vi "calc_drift.vi"(8 "error in (no error)":errorcluster caption="错误输入（无错误）", 11 "OneMotion 输入":refnum<class "OneMotion.lvclass">) -> (0 "error out":errorcluster caption="错误输出", 3 "OneMotion 输出":refnum<class "OneMotion.lvclass">)   [LabVIEW 2014, in "OneMotion.lvclass"]
uses:
  OneMotion.lvclass
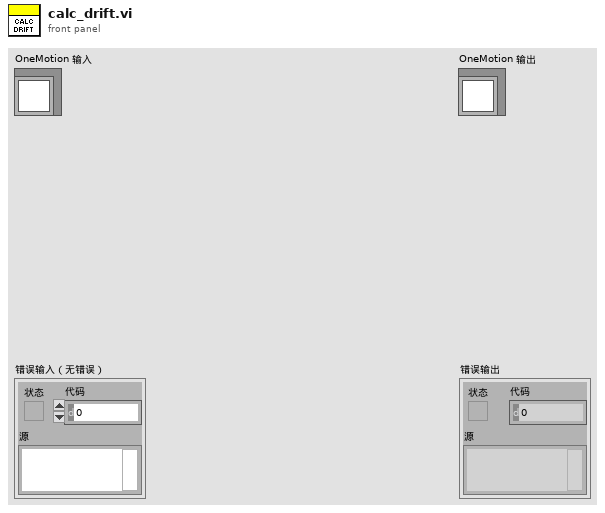
[diagram p1: front panel]
types:
  T1 = typedef "OneMotion.lvclass/backlash option.ctl" = enum16{"no backlash compensation", "compensation: from - to +", "compensation: from + to -"}
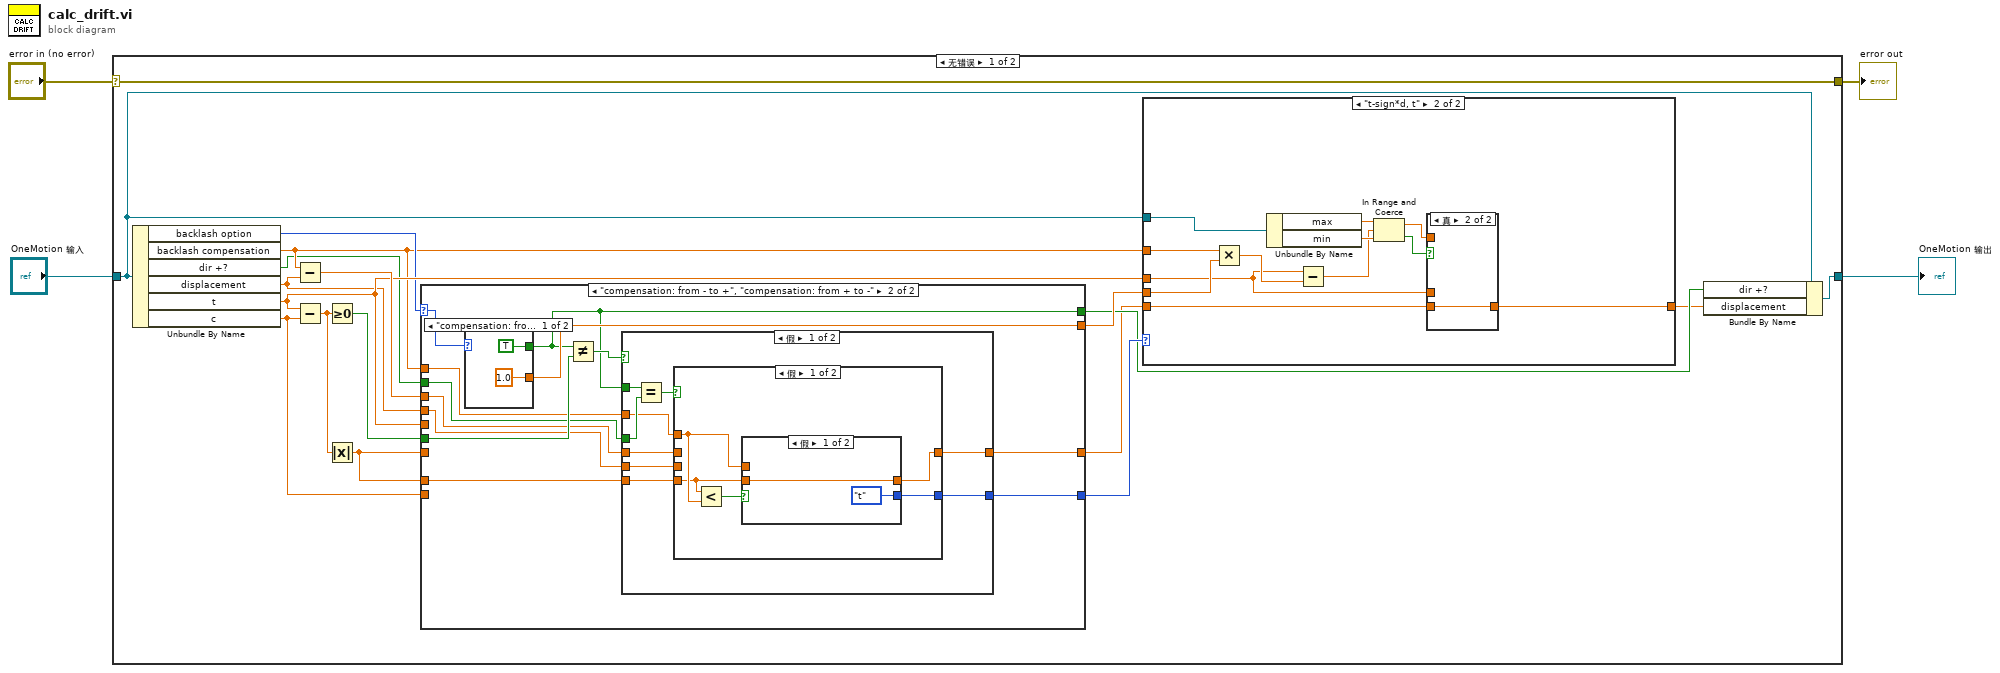
[diagram p0: block diagram]
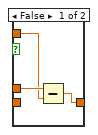
[diagram p3: hidden frame]
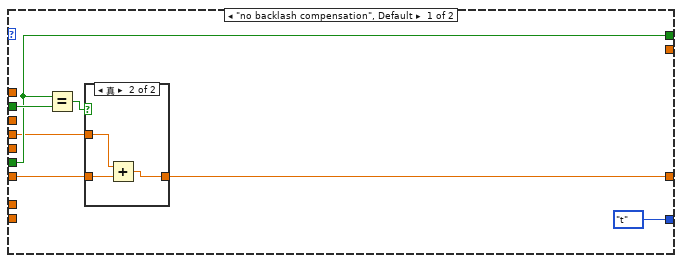
[diagram p4: hidden frame]
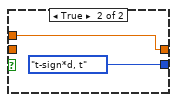
[diagram p6: hidden frame]
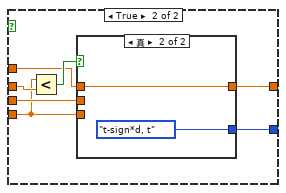
[diagram p7: hidden frame]
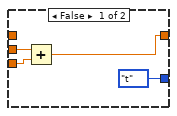
[diagram p8: hidden frame]
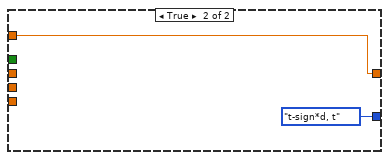
[diagram p9: hidden frame]
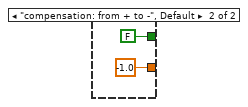
[diagram p10: hidden frame]
diagram:
  n1 = case shown="无错误" "error in (no error)" {
    selector: "error in (no error)" -> [w22 w101]
    tunnel: [w22 w101] -> w3
    tunnel: [w5 w100] -> w1
    tunnel: "OneMotion 输入" -> [w11 w100]
    frame No Error {
      n2 = Unbundle By Name(w11) -> ("backlash option"=w10:T1, "backlash compensation"=w9:dbl, "dir +?"=w7:bool, "displacement"=w6:dbl, "t"=w12:dbl, "c"=w8:dbl)
      n3 = Subtract(x=w9, y=w6) -> (x-y=w18:dbl)
      n4 = Subtract(x=w12, y=w8) -> (x-y=w21:dbl)
      n5 = Greater Or Equal To 0?(x=w21) -> (x >= 0?=w19:bool)
      n6 = Absolute Value(x=w21) -> (abs(x)=w16:dbl)
      n7 = case shown="\"compensation: from - to +\", \"compensation: from + to -\"" w10 {
        selector: w10 -> [_ w62]
        tunnel: w9 -> [_ w55]
        tunnel: w12 -> [_ _]
        tunnel: w8 -> [_ _]
        tunnel: [enum16{"t", "t-sign*d, t"}."t" w59] -> w20
        tunnel: w19 -> [w43 w60]
        tunnel: w7 -> [w45 w58]
        tunnel: w16 -> [_ w57]
        tunnel: w18 -> [_ w56]
        tunnel: [_ w54] -> w17
        tunnel: [w43 w53] -> w15
        tunnel: [w42 w52] -> w14
        tunnel: w16 -> [w41 _]
        tunnel: w6 -> [w40 w51]
        frame "no backlash compensation", Default {
          n8 = Equal?(x=w43, y=w45) -> (x = y?=w44:bool)
          n9 = case shown="真" w44 {
            tunnel: [w47 w50] -> w42
            tunnel: w41 -> [w47 w49]
            tunnel: w40 -> [_ w48]
            frame False {
            }
            frame True {
              n10 = Add(x=w48, y=w49) -> (x+y=w50:dbl)
            }
          }
        }
        frame "compensation: from - to +", "compensation: from + to -" {
          n11 = case shown="\"compensation: from - to +\"" w62 {
            tunnel: [1.0 -1.0] -> w54
            tunnel: [TRUE FALSE] -> w53
            frame "compensation: from - to +" {
            }
            frame "compensation: from + to -", Default {
            }
          }
          n12 = Not Equal?(x=w53, y=w60) -> (x != y?=w61:bool)
          n13 = case shown="假" w61 {
            tunnel: [w66 enum16{"t", "t-sign*d, t"}."t-sign*d, t"] -> w59
            tunnel: w58 -> [w70 _]
            tunnel: w53 -> [w69 _]
            tunnel: w57 -> [w68 _]
            tunnel: w56 -> [w67 _]
            tunnel: w55 -> [w65 w94]
            tunnel: [w64 w94] -> w52
            tunnel: w51 -> [w63 _]
            frame False {
              n14 = Equal?(x=w69, y=w70) -> (x = y?=w71:bool)
              n15 = case shown="假" w71 {
                tunnel: w68 -> [w72 w81]
                tunnel: w67 -> [_ w86]
                tunnel: [w75 w85] -> w66
                tunnel: w65 -> [w74 w84]
                tunnel: [w73 w83] -> w64
                tunnel: w63 -> [_ w82]
                frame False {
                  n16 = Less?(x=w72, y=w74) -> (x < y?=w76:bool)
                  n17 = case shown="假" w76 {
                    tunnel: [enum16{"t", "t-sign*d, t"}."t" enum16{"t", "t-sign*d, t"}."t-sign*d, t"] -> w75
                    tunnel: w74 -> [_ w79]
                    tunnel: [w77 w79] -> w73
                    tunnel: w72 -> [w77 _]
                    frame False {
                    }
                    frame True {
                    }
                  }
                }
                frame True {
                  n18 = Less?(x=w81, y=w86) -> (x < y?=w87:bool)
                  n19 = case shown="真" w87 {
                    tunnel: [enum16{"t", "t-sign*d, t"}."t" enum16{"t", "t-sign*d, t"}."t-sign*d, t"] -> w85
                    tunnel: w84 -> [_ w92]
                    tunnel: [w88 w92] -> w83
                    tunnel: w82 -> [w90 _]
                    tunnel: w81 -> [w89 _]
                    frame False {
                      n20 = Add(x=w90, y=w89) -> (x+y=w88:dbl)
                    }
                    frame True {
                    }
                  }
                }
              }
            }
            frame True {
            }
          }
        }
      }
      n21 = case shown="\"t-sign*d, t\"" w20 {
        tunnel: w11 -> [_ w30]
        tunnel: w12 -> [_ w26]
        tunnel: w9 -> [_ w35]
        tunnel: w17 -> [_ w34]
        tunnel: [w23 w25] -> w13
        tunnel: w14 -> [w23 w24]
        frame "t", Default {
        }
        frame "t-sign*d, t" {
          n22 = Multiply(x=w35, y=w34) -> (x*y=w33:dbl)
          n23 = Unbundle By Name(w30) -> ("max"=w32:dbl, "min"=w31:dbl)
          n24 = Subtract(x=w26, y=w33) -> (x-y=w27:dbl)
          n25 = In Range and Coerce(upper limit=w32, x=w27, lower limit=w31) -> (coerced(x)=w28:dbl, In Range?=w29:bool)
          n26 = case shown="真" w29 {
            tunnel: w28 -> [w37 _]
            tunnel: w26 -> [w38 _]
            tunnel: [w36 w39] -> w25
            tunnel: w24 -> [_ w39]
            frame False {
              n27 = Subtract(x=w38, y=w37) -> (x-y=w36:dbl)
            }
            frame True {
            }
          }
        }
      }
      n28 = Bundle By Name(cluster=w11, "dir +?"=w15, "displacement"=w13) -> (w5:refnum<class "OneMotion.lvclass">)
    }
    frame Error {
    }
  }
  "error out" <- w3
  "OneMotion 输出" <- w1
